vi "From Variant.vi"(8 "Error In":errorcluster, 10 "Variant":variant, 11 "TD Bool A In":refnum<class "1D Bool.lvclass">) -> (0 "Error Out":errorcluster, 3 "TD Bool A Out":refnum<class "1D Bool.lvclass">)   [LabVIEW 2017, in "Tree API.lvlib" / "1D Bool.lvclass"]
doc: "Dynamic dispatch interface for conversion of variant LV data to Tree Data classes."
uses:
  1D Bool.lvclass
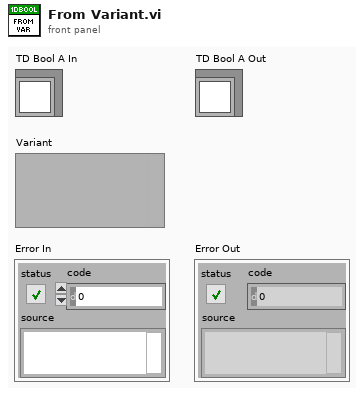
[diagram p1: front panel]
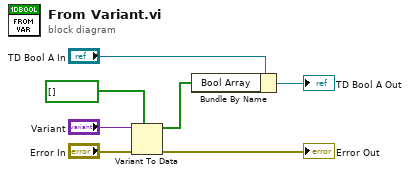
[diagram p0: block diagram]
diagram:
  n1 = Variant To Data(error in="Error In", type=bool[] [] ("Bool Array"), Variant="Variant") -> (data=w3:bool[], error out=→"Error Out":errorcluster)
  n2 = Bundle By Name(cluster="TD Bool A In", "Bool Array"=w3) -> (→"TD Bool A Out":refnum<class "1D Bool.lvclass">)
